vi "From Variant.vi"(8 "error in (no error)":errorcluster, 11 "Variant":variant) -> (0 "error out":errorcluster, 3 "Boolean out":refnum<class "Assertion 1D.lvclass">)   [LabVIEW 2020, in "Assertion 1D.lvclass"]
uses:
  <vilib>/gpm_packages/@cs/data-type-serializer/source/Assertion 1D/Assertion 1D.lvclass
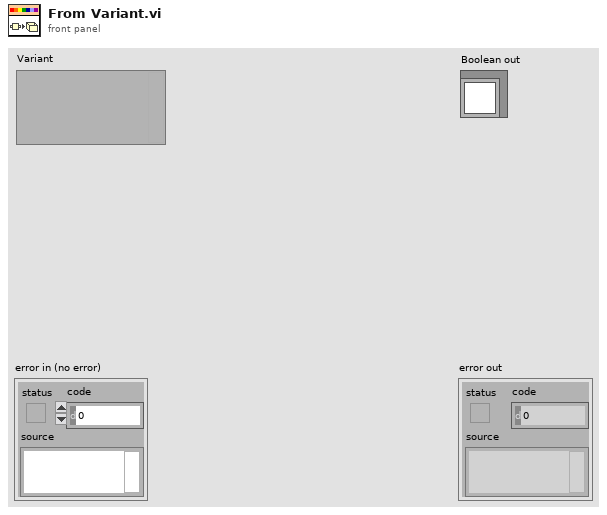
[diagram p1: front panel]
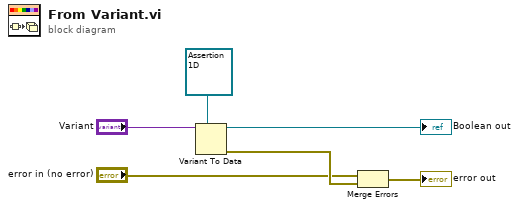
[diagram p0: block diagram]
diagram:
  n1 = Variant To Data(type=refnum<class "Assertion 1D.lvclass"> refnum ("Boolean in"), Variant="Variant") -> (data=→"Boolean out":refnum<class "Assertion 1D.lvclass">, error out=w5:errorcluster)  [unwired: 1 in]
  n2 = Merge Errors("error in (no error)", w5) -> (→"error out":errorcluster)
